vi "Write Verify Server.vi"(8 "error in (no error)":errorcluster, 10 "Verify Server":bool=TRUE, 11 "REST Client_JKI in":refnum<class "REST Client_JKI.lvclass">) -> (0 "error out":errorcluster, 3 "REST Client_JKI out":refnum<class "REST Client_JKI.lvclass">)   [LabVIEW 2018, in "REST Client.lvlib" / "REST Client_JKI.lvclass"]
doc: "Write Verify Server"
uses:
  REST Client_JKI.lvclass
  REST Client/REST Client.lvclass
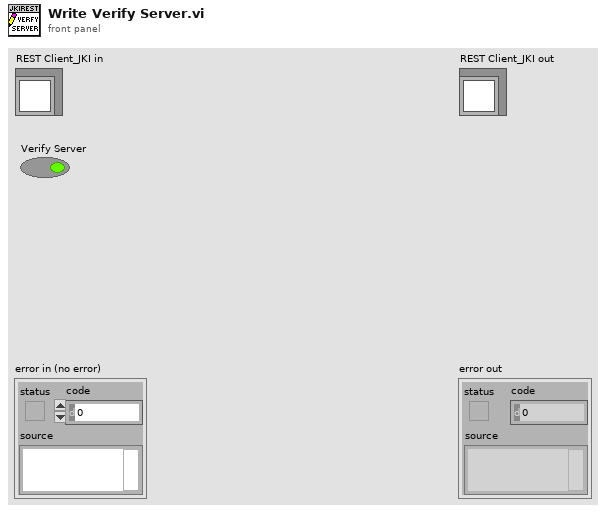
[diagram p1: front panel]
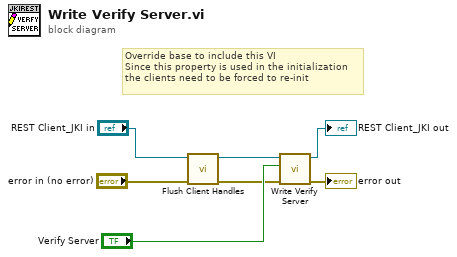
[diagram p0: block diagram]
diagram:
  # "Override base to include this VI\nSince this property is used in the initialization\nthe clients need to be forced to re-init"
  n1 = call-dynamic "Flush Client Handles.vi"("error in (no error)"="error in (no error)", "REST Client in"="REST Client_JKI in") -> ("error out"=w3:errorcluster, "REST Client out"=w1:refnum<class "REST Client_JKI.lvclass">)  [unwired: 8 in]
  n2 = call-parent "Write Verify Server.vi"("error in (no error)"=w3, "Verify Server"="Verify Server", "REST Client in"=w1) -> ("error out"=→"error out":errorcluster, "REST Client out"=→"REST Client_JKI out":refnum<class "REST Client_JKI.lvclass">)  [unwired: 7 in]
